vi "AT_ErrorCodeHandler.vi"(0 "Error":i32, 1 "Feature Name":string) -> (7 "error out":errorcluster)   [LabVIEW 2019]
doc: "Error Code Handler\n\nOutput:\n void\n\nInput:\n I32 Error\n String Feature name\n\nInterprets andor error codes and determines wether a dll function call was successfull or not."
panel:
  out "Error Code Enum":i32(ring) items=["SUCCESS", "NOT INITIALISED", "NOT IMPLEMENTED", "READ ONLY", "NOT READABLE", "NOT WRITABLE", "OUT OF RANGE", "INDEX NOT AVAILABLE", "INDEX NOT IMPLEMENTED", "EXCEEDED MAX STRING LENGTH", "CONNECTION", "NO DATA", "INVALID HANDLE", "TIMED OUT", "BUFFER FULL", "INVALID SIZE", "INVALID ALIGNMENT", "COMM", "STRING NOT AVAILABLE", "STRING NOT IMPLEMENTED", "NULL FEATURE", "NULL HANDLE", "NULL IMPLEMENTED VAR", "NULL READABLE VAR", "NULL READONLY VAR", "NULL WRITABLE VAR", "NULL MIN VALUE", "NULL MAX VALUE", "NULL VALUE", "NULL STRING", "NULL COUNT VAR", "NULL IS AVAILABLE VAR", "NULL MAX STRING LENGTH", "NULL EV CALL BACK", "NULL QUEUE POINTER", "NULL WAIT POINTER", "NULL POINTER SIZE", "NO MEMORY", "DEVICE IN USE"]
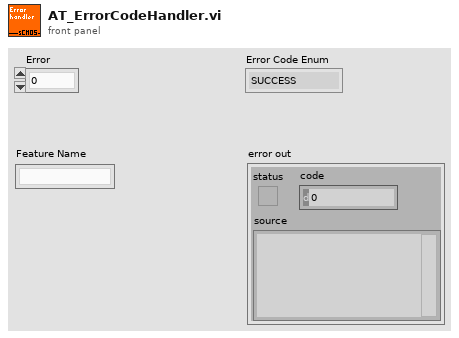
[diagram p1: front panel]
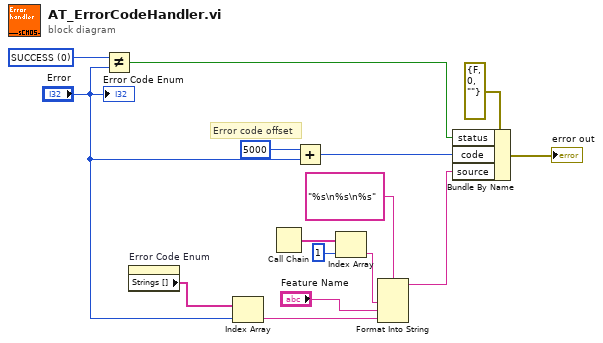
[diagram p0: block diagram]
diagram:
  w7 = 0 items=["SUCCESS", "NOT INITIALISED", "NOT IMPLEMENTED", "READ ONLY", "NOT READABLE", "NOT WRITABLE", "OUT OF RANGE", "INDEX NOT AVAILABLE", "INDEX NOT IMPLEMENTED", "EXCEEDED MAX STRING LENGTH", "CONNECTION", "NO DATA", "INVALID HANDLE", "TIMED OUT", "BUFFER FULL", "INVALID SIZE", "INVALID ALIGNMENT", "COMM", "STRING NOT AVAILABLE", "STRING NOT IMPLEMENTED", "NULL FEATURE", "NULL HANDLE", "NULL IMPLEMENTED VAR", "NULL READABLE VAR", "NULL READONLY VAR", "NULL WRITABLE VAR", "NULL MIN VALUE", "NULL MAX VALUE", "NULL VALUE", "NULL STRING", "NULL COUNT VAR", "NULL IS AVAILABLE VAR", "NULL MAX STRING LENGTH", "NULL EV CALL BACK", "NULL QUEUE POINTER", "NULL WAIT POINTER", "NULL POINTER SIZE", "NO MEMORY", "DEVICE IN USE"] ("Error Codes")
  # "Error code offset"
  n1 = Not Equal?(x=w7, y="Error") -> (x != y?=w11:bool)
  n2 = property on="Error Code Enum" class="Ring (strict)"() -> ("Strings []"=w6:string[])  [unwired: 2 in, 2 out]
  n3 = Index Array(array=w6, index="Error") -> (element=w1:string)
  n4 = Call Chain() -> (call chain=w14:string[])
  n5 = Add(x=5000, y="Error") -> (x+y=w10:i32)
  n6 = Index Array(array=w14, index=1) -> (element=w15:string)
  n7 = Format Into String(format string="%s\n%s\n%s", w15, "Feature Name", w1) -> (resulting string=w9:string)  [unwired: 2 in, 1 out]
  n8 = Bundle By Name(cluster=errorcluster {"status"=FALSE, "code"=0, "source"=""} ("error constant"), "status"=w11, "code"=w10, "source"=w9) -> (→"error out":errorcluster)
  "Error Code Enum" <- "Error"
